vi "get_instances.vi"(8 "error in (no error)":errorcluster, 10 "Base Class (LabVIEW Object)":refnum<class>, 11 "Default Lookup in":refnum<class "Default Lookup.lvclass">) -> (0 "error out":errorcluster, 2 "instances":refnum<data-value>[](array[refnum]), 3 "Default Lookup out":refnum<class "Default Lookup.lvclass">)   [LabVIEW 2014, in "LVCOOOP.lvlib" / "Lookup API.lvlib" / "Default Lookup.lvclass"]
uses:
  Default Lookup.lvclass
  Default Lookup.lvclass/Default Lookup.ctl
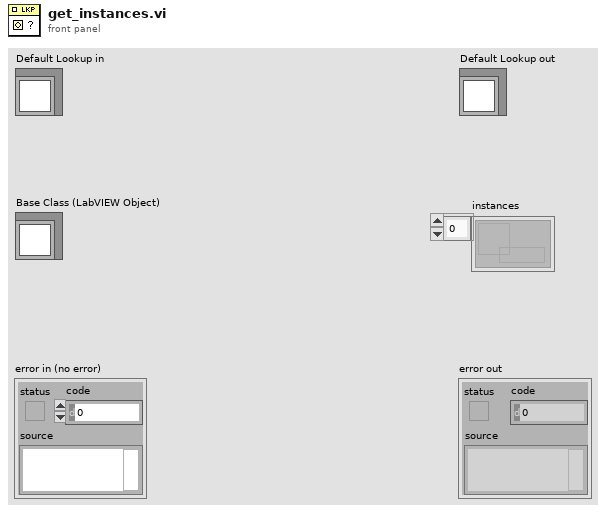
[diagram p1: front panel]
types:
  T1 = typedef "LVCOOOP.lvlib/Lookup API.lvlib/Default Lookup.lvclass/lookup_data.ctl" = cluster{"instances":refnum<data-value>[], "listeners":refnum<user-event>[]}
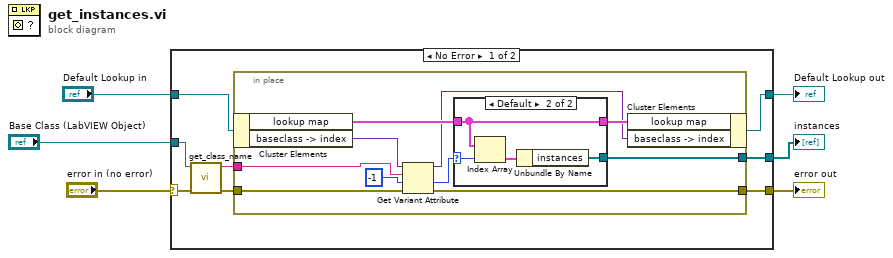
[diagram p0: block diagram]
diagram:
  n1 = case shown="No Error" "error in (no error)" {
    selector: "error in (no error)" -> [w14 w31]
    tunnel: [w7 w31] -> w5
    tunnel: "Base Class (LabVIEW Object)" -> [w13 _]
    tunnel: "Default Lookup in" -> [w12 w30]
    tunnel: [w9 _] -> w2
    tunnel: [w8 w30] -> w1
    frame No Error {
      n2 = call "get_class_name.vi"("error in (no error)"=w14, "LabVIEW Object in"=w13) -> ("error out"=w10:errorcluster, "class name"=w11:string)  [unwired: 8 in]
      n3 = in-place {
        in-place-border: w11 -> [w23]
        in-place-border: w10 -> [w21]
        in-place-border: [w16] -> w9
        in-place-border: [w15] -> w7
        n4 = in-place-cluster #1(w12) -> ("lookup map"=w19:T1[], "baseclass -> index"=w24:variant)
        n5 = Get Variant Attribute(Variant=w24, name=w23, default value (empty Variant)=-1, error in=w21) -> (duplicate Variant=w17:variant, value=w20:i32, error out=w15:errorcluster)  [unwired: 1 out]
        n6 = case shown="Default" w20 {
          selector: w20 -> [_ w29]
          tunnel: w19 -> [w25 w26]
          tunnel: [w25 w26] -> w18
          tunnel: [_ w27] -> w16
          frame -1 {
          }
          frame Default {
            n7 = Index Array(array=w26, index=w29) -> (element=w28:T1)
            n8 = Unbundle By Name(w28) -> ("instances"=w27:refnum<data-value>[])
          }
        }
        n9 = in-place-cluster #1("lookup map"=w18, "baseclass -> index"=w17) -> (w8:refnum<class "Default Lookup.lvclass">)
      }
    }
    frame Error {
    }
  }
  "error out" <- w5
  "Default Lookup out" <- w1
  "instances" <- w2
